vi "CRYTable Value Delete.vi"(7 "TableVI":refnum<vi>, 8 "Index Down":i32, 9 "Type Down":enum16{"Curves", "Values", "Results", "WFM"}(ring), 10 "Index Up":i32, 11 "Type Up":enum16{"Curves", "Values", "Results", "WFM"}(ring)) -> ()   [LabVIEW 2013]
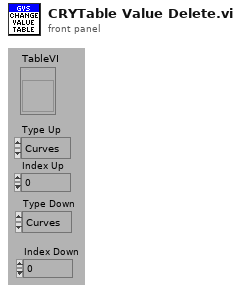
[diagram p1: front panel]
types:
  T1 = typedef "LVRowAndColumnTypeDef.ctl" = cluster{"Row":i32, "Column":i32}
  T2 = typedef "CRYData Cluster.ctl" = cluster{"Name":string, "Curve":cluster{"x":dbl, "y":dbl, "z":dbl}[], "X data":u16, "Y data":u16, "Z data":u16, "X axis":u16, "Y axis":u16, "Z axis":u16, "X unit":string, "Y unit":string, "Z unit":string, "X dB ref":dbl, "Y dB ref":dbl, "Z dB ref":dbl, "single val":bool, "protected":bool, "display X":bool, "display Y":bool, "display Z":bool, "Test Info":string, "Step No.":i32, "Plot Settings":cluster{"Color":u32, "Interpolation":u8, "Point Style":u8, "Line Style":u8, "Point Color":u32, "Line Width":u8, "Bar Plot Style":u8, "Fill To":i16}, "AutoProtect":bool}
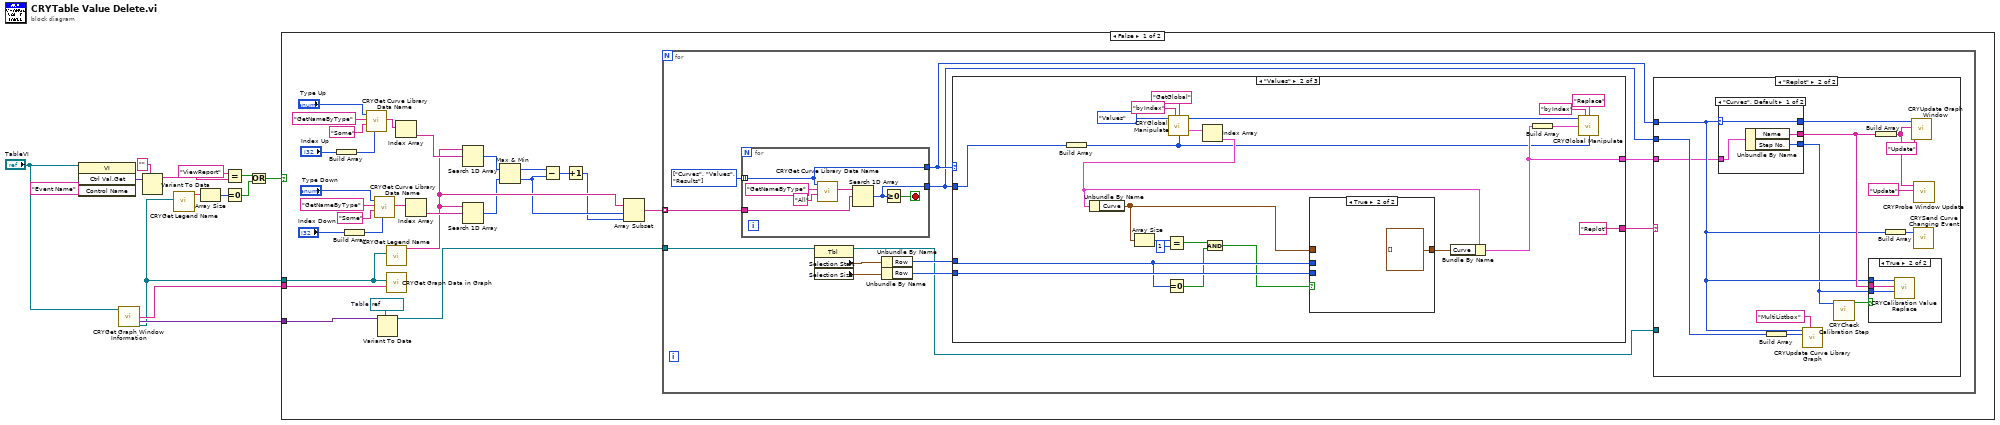
[diagram p0: block diagram]
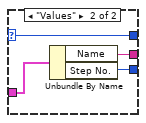
[diagram p4: hidden frame]
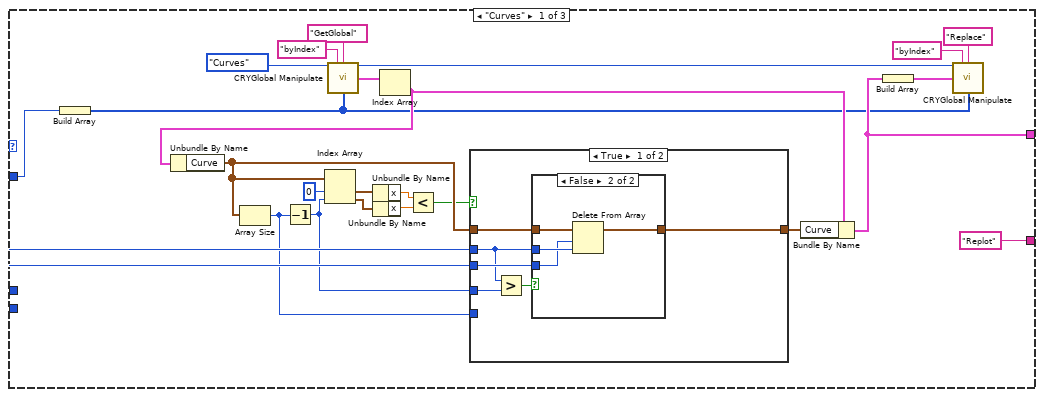
[diagram p5: hidden frame]
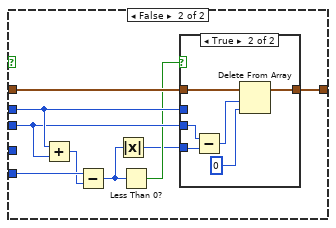
[diagram p7: hidden frame]
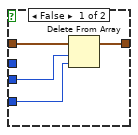
[diagram p8: hidden frame]
diagram:
  n1 = invoke class="VI" method="Ctrl Val.Get"(reference="TableVI", "Control Name"="Event Name") -> ("Get Control Value Variant"=w12:variant)  [unwired: 2 in, 3 out]
  n2 = call "CRYGet Graph Window Information.vi"("pGraph VI In"="TableVI") -> ("Graph Type Out"=w5:string, "Graph Control Ref Out"=w14:variant, "Legend Ref Out"=w4:refnum<vi>)  [unwired: 4 in, 8 out]
  n3 = Variant To Data(type="" ("Control Name"), Variant=w12) -> (data=w9:string)  [unwired: 1 in, 1 out]
  n4 = call "CRYGet Legend Name.vi"("MCListbox Refnum"=w4) -> ("Names Out"=w7:string[])  [unwired: 10 in]
  n5 = Array Size(array=w7) -> (size(s)=w6:i32)
  n6 = Equal?(x="ViewReport", y=w9) -> (x = y?=w2:bool)
  n7 = Equal To 0?(x=w6) -> (x = 0?=w1:bool)
  n8 = Or(x=w2, y=w1) -> (x .or. y?=w3:bool)
  n9 = case shown="False" w3 {
    tunnel: w14 -> [w40 _]
    tunnel: w5 -> [w39 _]
    tunnel: w4 -> [w38 _]
    frame False {
      w41 = refnum<vi> refnum  # Table
      n10 = Build Array("Index Up") -> (w33:i32[])
      n11 = Build Array("Index Down") -> (w28:i32[])
      n12 = call "CRYGet Curve Library Data Name.vi"("nData"=w33, "sOption"="Some", "sAction"="GetNameByType", "Type"="Type Up") -> ("sNames"=w25:string[])  [unwired: 4 in, 3 out]
      n13 = call "CRYGet Curve Library Data Name.vi"("nData"=w28, "sOption"="Some", "sAction"="GetNameByType", "Type"="Type Down") -> ("sNames"=w23:string[])  [unwired: 4 in, 3 out]
      n14 = Variant To Data(type=w41, Variant=w40) -> (data=w36:refnum<vi>)  [unwired: 1 in, 1 out]
      n15 = call "CRYGet Legend Name.vi"("MCListbox Refnum"=w38) -> ("Names Out"=w21:string[])  [unwired: 10 in]
      n16 = call "CRYGet Graph Data in Graph.vi"("Graph Type"=w39, "Legend Refnum"=w38) -> ()  [unwired: 2 in, 8 out]
      n17 = Index Array(array=w25) -> (element=w24:string)  [unwired: 1 in]
      n18 = Index Array(array=w23) -> (element=w22:string)  [unwired: 1 in]
      n19 = Search 1D Array(1D array=w21, element=w24) -> (index of element=w19:i32)  [unwired: 1 in]
      n20 = Search 1D Array(1D array=w21, element=w22) -> (index of element=w18:i32)  [unwired: 1 in]
      n21 = Max & Min(x=w19, y=w18) -> (max(x,y)=w20:i32, min(x,y)=w17:i32)
      n22 = Subtract(x=w20, y=w17) -> (x-y=w16:i32)
      n23 = Increment(x=w16) -> (x+1=w15:i32)
      n24 = Array Subset(array=w21, index=w17, length=w15) -> (w37:string[])
      n25 = for {
        tunnel: w37 -> [w52] mode=indexing
        tunnel: w36 -> [w47]
        w53 = enum16{"Curves", "Values", "Results", "WFM"}[] [enum."Curves", enum."Values", enum."Results"] items=["Curves", "Values", "Results", "WFM"]
        n26 = for {
          tunnel: w53 -> [w158] mode=indexing
          tunnel: w52 -> [w159]
          tunnel: [w158] -> w45
          tunnel: [w157] -> w44
          stop <- w160 stop-if-true
          n27 = call "CRYGet Curve Library Data Name.vi"("sOption"="All", "sAction"="GetNameByType", "Type"=w158) -> ("sNames"=w161:string[])  [unwired: 5 in, 3 out]
          n28 = Search 1D Array(1D array=w161, element=w159) -> (index of element=w157:i32)  [unwired: 1 in]
          n29 = Greater Or Equal To 0?(x=w157) -> (x >= 0?=w160:bool)
        }
        n30 = property class="Tbl"(reference=w47) -> (reference out=w43:refnum<vi>, "Selection Start"=w50:T1, "Selection Size"=w51:T1)  [unwired: 1 in, 1 out]
        n31 = Unbundle By Name(w50) -> ("Row"=w49:i32)
        n32 = Unbundle By Name(w51) -> ("Row"=w48:i32)
        n33 = case shown="\"Values\"" w45 {
          tunnel: ["Replot" ("output string") "Replot" ("output string") _] -> w46
          tunnel: w44 -> [w89 w140 _]
          tunnel: w49 -> [w94 w150 _]
          tunnel: w48 -> [w93 w151 _]
          tunnel: [w83 w138 _] -> w42
          frame "Curves" {
            n34 = Build Array(w89) -> (w78:i32[])
            n35 = call "CRYGlobal Manipulate.vi"("Type"=enum16{"Curves", "Values", "Results", "WFM"}."Curves", "sOption"="byIndex", "sAction"="GetGlobal", "nData"=w78) -> ("Type out"=w85:enum16{"Curves", "Values", "Results", "WFM"}, "Curves Out"=w88:T2[])  [unwired: 5 in, 5 out]
            n36 = Index Array(array=w88) -> (element=w87:T2)  [unwired: 1 in]
            n37 = Unbundle By Name(w87) -> ("Curve"=w96:cluster{"x":dbl, "y":dbl, "z":dbl}[])
            n38 = Array Size(array=w96) -> (size(s)=w90:i32)
            n39 = Decrement(x=w90) -> (x-1=w91:i32)
            n40 = Index Array(array=w96, index #1=0 ("index"), index #2=w91) -> (element #1=w100:cluster{"x":dbl, "y":dbl, "z":dbl}, element #2=w99:cluster{"x":dbl, "y":dbl, "z":dbl})
            n41 = Unbundle By Name(w100) -> ("x"=w98:dbl)
            n42 = Unbundle By Name(w99) -> ("x"=w97:dbl)
            n43 = Less?(x=w98, y=w97) -> (x < y?=w92:bool)
            n44 = case shown="True" w92 {
              tunnel: w96 -> [w108 w122]
              tunnel: [w107 w121] -> w95
              tunnel: w93 -> [w106 w119]
              tunnel: w94 -> [w105 w120]
              tunnel: w91 -> [w104 _]
              tunnel: w90 -> [_ w118]
              frame True {
                n45 = Greater?(x=w105, y=w104) -> (0:w103:bool)
                n46 = case shown="False" w103 {
                  tunnel: w105 -> [_ w113]
                  tunnel: w106 -> [_ w112]
                  tunnel: w108 -> [w109 w111]
                  tunnel: [w109 w110] -> w107
                  frame True {
                  }
                  frame False {
                    n47 = Delete From Array(array=w111, length=w112, index=w113) -> (array with subset deleted=w110:cluster{"x":dbl, "y":dbl, "z":dbl}[])  [unwired: 1 out]
                  }
                }
              }
              frame False {
                n48 = Add(x=w120, y=w119) -> (x+y=w117:i32)
                n49 = Subtract(x=w118, y=w117) -> (x-y=w116:i32)
                n50 = Absolute Value(x=w116) -> (abs(x)=w114:i32)
                n51 = Less Than 0?(x=w116) -> (x < 0?=w115:bool)
                n52 = case shown="True" w115 {
                  tunnel: w120 -> [_ _]
                  tunnel: w119 -> [w126 w129]
                  tunnel: w122 -> [w125 w132]
                  tunnel: [w124 w131] -> w121
                  tunnel: w114 -> [w123 w128]
                  frame False {
                    n53 = Delete From Array(array=w125, length=w126, index=w123) -> (array with subset deleted=w124:cluster{"x":dbl, "y":dbl, "z":dbl}[])  [unwired: 1 out]
                  }
                  frame True {
                    n54 = Subtract(x=w129, y=w128) -> (x-y=w127:i32)
                    n55 = Delete From Array(array=w132, length=w127, index=0) -> (array with subset deleted=w131:cluster{"x":dbl, "y":dbl, "z":dbl}[])  [unwired: 1 out]
                  }
                }
              }
            }
            n56 = Bundle By Name(cluster=w87, "Curve"=w95) -> (w83:T2)
            n57 = Build Array(w83) -> (w84:T2[])
            n58 = call "CRYGlobal Manipulate.vi"("Type"=w85, "sOption"="byIndex", "sAction"="Replace", "Curves"=w84, "nData"=w78) -> ()  [unwired: 4 in, 7 out]
          }
          frame "Values" {
            n59 = Build Array(w140) -> (w133:i32[])
            n60 = Equal To 0?(x=w150) -> (x = 0?=w146:bool)
            n61 = call "CRYGlobal Manipulate.vi"("Type"=enum16{"Curves", "Values", "Results", "WFM"}."Values", "sOption"="byIndex", "sAction"="GetGlobal", "nData"=w133) -> ("Type out"=w142:enum16{"Curves", "Values", "Results", "WFM"}, "Values Out"=w144:T2[])  [unwired: 5 in, 5 out]
            n62 = Index Array(array=w144) -> (element=w139:T2)  [unwired: 1 in]
            n63 = Unbundle By Name(w139) -> ("Curve"=w153:cluster{"x":dbl, "y":dbl, "z":dbl}[])
            n64 = Array Size(array=w153) -> (size(s)=w149:i32)
            n65 = Equal?(x=w149, y=1) -> (x = y?=w147:bool)
            n66 = And(x=w147, y=w146) -> (x .and. y?=w145:bool)
            n67 = case shown="True" w145 {
              tunnel: w153 -> [w155 _]
              tunnel: [w155 cluster{"x":dbl, "y":dbl, "z":dbl}[] [] ("Curve")] -> w152
              tunnel: w151 -> [_ _]
              tunnel: w150 -> [_ _]
              frame False {
              }
              frame True {
              }
            }
            n68 = Bundle By Name(cluster=w139, "Curve"=w152) -> (w138:T2)
            n69 = Build Array(w138) -> (w141:T2[])
            n70 = call "CRYGlobal Manipulate.vi"("Type"=w142, "sOption"="byIndex", "sAction"="Replace", "Curves"=w141, "nData"=w133) -> ()  [unwired: 4 in, 7 out]
          }
          frame "Results", Default {
          }
        }
        n71 = case shown="\"Replot\"" w46 {
          tunnel: w45 -> [_ w59]
          tunnel: w44 -> [_ w61]
          tunnel: w43 -> [_ _]
          tunnel: w42 -> [_ w54]
          frame Default {
          }
          frame "Replot" {
            n72 = case shown="\"Curves\", Default" w59 {
              selector: w59 -> [w72 w76]
              tunnel: [w73 w77] -> w62
              tunnel: [w72 w76] -> w65
              tunnel: [w71 w75] -> w55
              tunnel: w54 -> [w70 w74]
              frame "Curves", Default {
                n73 = Unbundle By Name(w70) -> ("Name"=w73:string, "Step No."=w71:i32)
              }
              frame "Values" {
                n74 = Unbundle By Name(w74) -> ("Name"=w77:string, "Step No."=w75:i32)
              }
            }
            n75 = Build Array(w61) -> (w58:i32[])
            n76 = call "CRYUpdate Curve Library Graph.vi"("sOption 1"="MultiListbox" ("sOption"), "Index"=w58, "Type"=w59) -> ()  [unwired: 9 in]
            n77 = call "CRYCheck Calibration Step.vi"("Step No"=w55) -> ("Is Calibration?"=w56:bool)  [unwired: 9 in, 1 out]
            n78 = case shown="True" w56 {
              tunnel: w59 -> [_ w69]
              tunnel: w62 -> [_ w68]
              tunnel: w55 -> [_ w67]
              frame False {
              }
              frame True {
                n79 = call "CRYCalibration Value Replace.vi"("Step No."=w67, "Corr/EQ/Sens Name"=w68, "Type"=w69) -> ()  [unwired: 9 in]
              }
            }
            n80 = Build Array(w62) -> (w64:string[])
            n81 = Build Array(w59) -> (w63:enum16{"Curves", "Values", "Results", "WFM"}[])
            n82 = call "CRYUpdate Graph Window.vi"("sOption"="Update", "Del/Update Names"=w64, "Type"=w65) -> ()  [unwired: 1 in, 8 out]
            n83 = call "CRYSend Curve Changing Event.vi"("Type"=w63) -> ()  [unwired: 11 out]
            n84 = call "CRYProbe Window Update.vi"("sAction"="Update", "Names"=w64) -> ()  [unwired: 2 in, 8 out]
          }
        }
      }
    }
    frame True {
    }
  }
